vi "kSAComm Connect.vi"(0 "IP Address":string="localhost") -> (2 "Connect":bool, 3 "kSAComm ref out":refnum<k24>)   [LabVIEW 2019]
uses:
  C:/Users/tim/Documents/kSAComm LabView Sample/kSACommInterface.dll
  kSACommInterface.dll
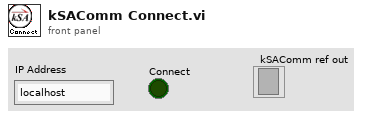
[diagram p1: front panel]
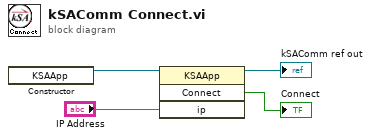
[diagram p0: block diagram]
diagram:
  n1 = constructor class="KSAApp"() -> (reference out=w1:refnum<k24>)  [unwired: 3 in, 2 out]
  n2 = invoke class="KSAApp" method="Connect"(reference=w1, "ip"="IP Address") -> (reference out=→"kSAComm ref out":refnum<k24>, "Connect"=→"Connect":bool)  [unwired: 2 in, 2 out]
